vi "Dispenser_Backup.vi"() -> ()   [LabVIEW 2016]
uses:
  <vilib>/Utility/file.llb/Read Delimited Spreadsheet (string).vi
  Other Models/EFD Ultimus V/EFD Ultimus V.lvlib
panel:
  out "error out":errorcluster
  out "String":string
  in  "VISA resource name":refnum<visa-resource-name>="COM1"
  in  "Serial Configuration":T1={"Baud Rate "=115200, "Parity "=0, "Data Bits "=8, "Stop Bits"=10} {"Stop Bits" items=["1.0"=10, "1.5"=15, "2.0"=20]; "Data Bits" items=["7"=7, "8"=8]; "Parity" items=["None", "Odd", "Even"]; "Baud Rate" items=["9600"=9600, "19200"=19200, "38400"=38400, "115200"=115200]}
  in  "Z":dbl format="%#_13g"
  in  "Y":dbl format="%#_13g"
  in  "X":dbl format="%#_13g"
  in  "Path":path
  # "Origin"
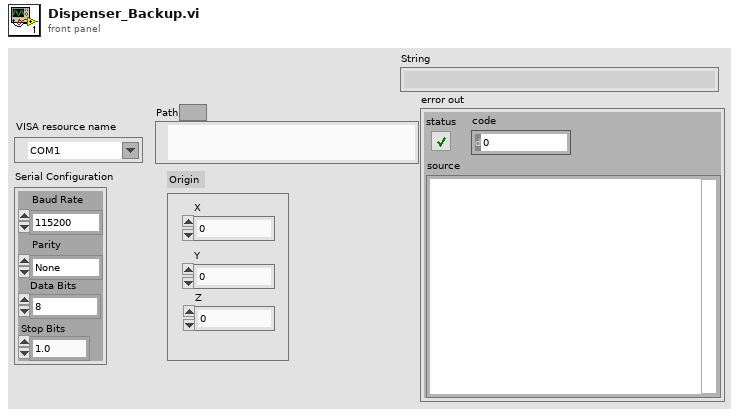
[diagram p1: front panel]
types:
  T1 = cluster{"Baud Rate ":u32, "Parity ":u16, "Data Bits ":u16, "Stop Bits":u16}
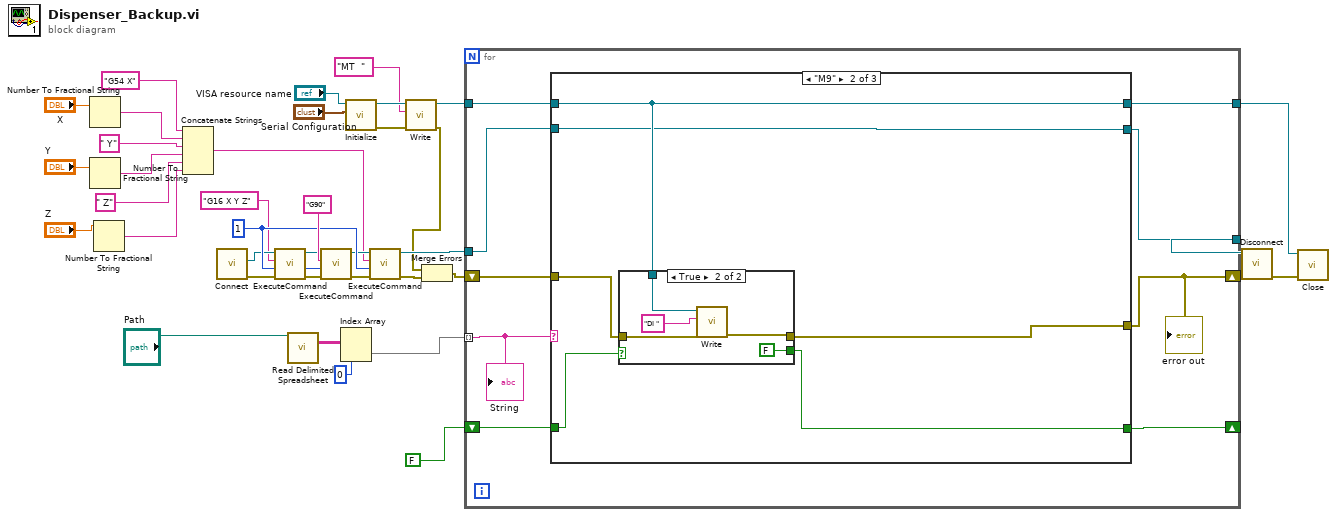
[diagram p0: block diagram]
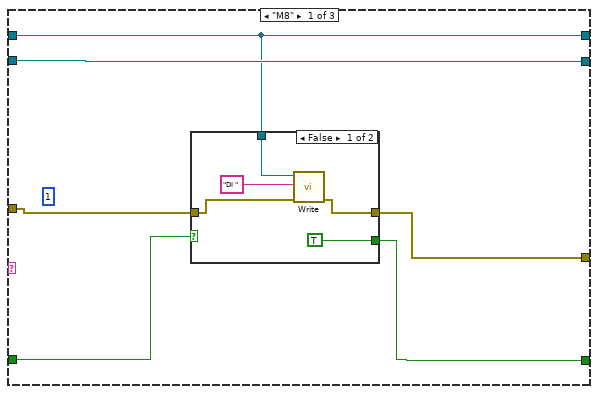
[diagram p2: hidden frame]
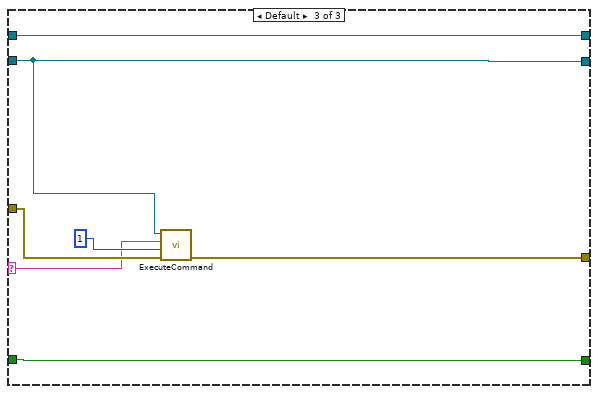
[diagram p5: hidden frame]
diagram:
  w29 = 1
  n1 = Number To Fractional String(number="X") -> (F-format string=w11:string)  [unwired: 3 in]
  n2 = Number To Fractional String(number="Y") -> (F-format string=w13:string)  [unwired: 3 in]
  n3 = Number To Fractional String(number="Z") -> (F-format string=w15:string)  [unwired: 3 in]
  n4 = Concatenate Strings("G54 X", w11, " Y", w13, " Z", w15) -> (w9:string)
  n5 = call "Connect.vi"() -> ("error out"=w32:errorcluster, "controller"=w7:refnum<k24>)  [unwired: 10 in]
  n6 = call "ExecuteCommand.vi"("Command Code"="G16 X Y Z", "controller in"=w7) -> ("controller out"=w8:refnum<k24>)  [unwired: 7 in, 2 out]
  n7 = call-poly <vilib>:"Read Delimited Spreadsheet.vi"("file path (dialog if empty)"="Path") -> ("all rows"=w36:string[][])  [unwired: 9 in, 5 out]
  n8 = call "ExecuteCommand.vi"("error in (no error)"=w32, "taskId"=w29, "Command Code"="G90", "controller in"=w8) -> ("error out"=w30:errorcluster, "controller out"=w28:refnum<k24>)  [unwired: 5 in, 1 out]
  n9 = Index Array(array=w36, index (col)=0) -> (element=w33:string[])  [unwired: 1 in]
  n10 = call "Initialize.vi"("Serial Configuration"="Serial Configuration", "VISA resource name"="VISA resource name") -> ("error out"=w4:errorcluster, "VISA resource name out"=w3:refnum<visa-resource-name>)  [unwired: 8 in]
  n11 = call "ExecuteCommand.vi"("error in (no error)"=w30, "taskId"=w29, "Command Code"=w9, "controller in"=w28) -> ("error out"=w24:errorcluster, "controller out"=w27:refnum<k24>)  [unwired: 5 in, 1 out]
  n12 = call "Write.vi"("error in (no error)"=w4, "Command To Write"="MT  ", "VISA resource name"=w3) -> ("error out"=w1:errorcluster, "VISA resource name out"=w5:refnum<visa-resource-name>)  [unwired: 7 in]
  n13 = Merge Errors(w1, w24) -> (w23:errorcluster)
  n14 = for {
    tunnel: w33 -> [w42] mode=indexing
    shift-right: [w46] -> w22
    shift-left: w23 -> [w40]
    shift-right: [w43] -> _
    shift-left: FALSE -> [w44]
    tunnel: w27 -> [w41]
    tunnel: [w45] -> w21
    tunnel: w5 -> [w39]
    tunnel: [w38] -> w19
    n15 = case shown="\"M9\"" w42 {
      selector: w42 -> [_ _ w73]
      tunnel: w40 -> [w47 w65 w79]
      tunnel: w41 -> [w52 w60 w74]
      tunnel: [w51 w61 w78] -> w46
      tunnel: [w52 w60 w74] -> w45
      tunnel: w44 -> [w50 w64 w76]
      tunnel: [w49 w63 w76] -> w43
      tunnel: w39 -> [w48 w62 w75]
      tunnel: [w48 w62 w75] -> w38
      frame "M8" {
        (unwired) 1
        n16 = case shown="False" w50 {
          selector: w50 -> [_ w58]
          tunnel: w47 -> [w55 w59]
          tunnel: [w54 w59] -> w51
          tunnel: [TRUE w58] -> w49
          tunnel: w48 -> [w56 _]
          frame False {
            n17 = call "Write.vi"("error in (no error)"=w55, "Command To Write"="DI ", "VISA resource name"=w56) -> ("error out"=w54:errorcluster)  [unwired: 7 in, 1 out]
          }
          frame True {
          }
        }
      }
      frame "M9" {
        n18 = case shown="True" w64 {
          selector: w64 -> [w66 _]
          tunnel: w65 -> [w67 w71]
          tunnel: [w67 w70] -> w61
          tunnel: [w66 FALSE] -> w63
          tunnel: w62 -> [_ w69]
          frame False {
          }
          frame True {
            n19 = call "Write.vi"("error in (no error)"=w71, "Command To Write"="DI ", "VISA resource name"=w69) -> ("error out"=w70:errorcluster)  [unwired: 7 in, 1 out]
          }
        }
      }
      frame Default {
        n20 = call "ExecuteCommand.vi"("error in (no error)"=w79, "taskId"=1, "Command Code"=w73, "controller in"=w74) -> ("error out"=w78:errorcluster)  [unwired: 5 in, 2 out]
      }
    }
    "error out" <- w46
    "String" <- w42
  }
  n21 = call "Disconnect.vi"("error in (no error)"=w22, "controller"=w21) -> ("error out"=w20:errorcluster)  [unwired: 9 in]
  n22 = call "Close.vi"("error in (no error)"=w20, "VISA resource name"=w19) -> ()  [unwired: 9 in, 1 out]
